vi "wireVI.vi"() -> ()   [LabVIEW 2013]
panel:
  out "Output Pulse":dbl[][](array[numeric])
  in  "Input Pulse":dbl[][](array[numeric])
  in  "Wire Length (m)":dbl
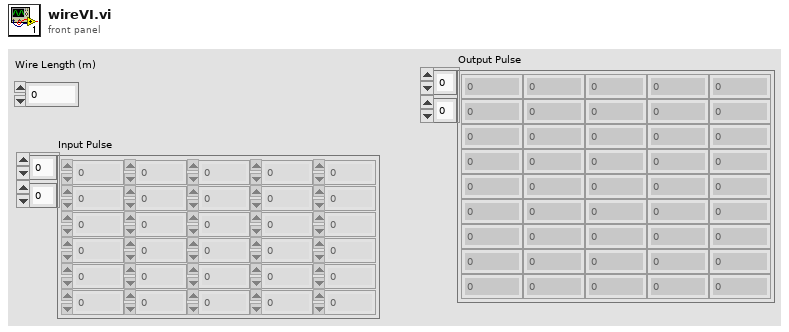
[diagram p1: front panel]
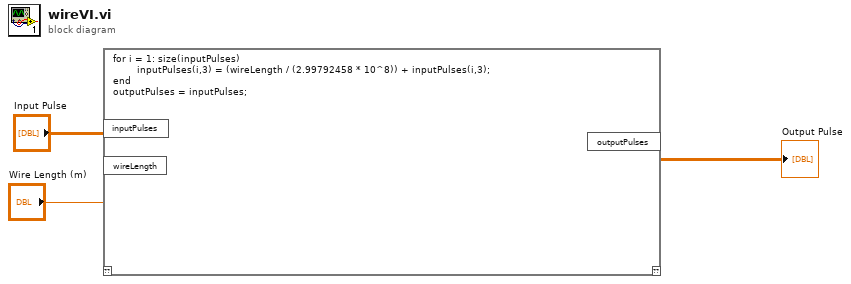
[diagram p0: block diagram]
diagram:
  n1 = script code="for i = 1: size(inputPulses)\n        inputPulses(i,3) = (wireLength / (2.99792458 * 10^8)) + inputPulses(i,3);\nend \noutputPulses = inputPulses;"("inputPulses"="Input Pulse", "wireLength"="Wire Length (m)") -> ("outputPulses"=→"Output Pulse":dbl[][])  [unwired: 1 in, 1 out]
